vi "NI VeriStand - Create and Load Runtime Configuration File.vi"(6 "File Path":string, 7 "Version":string, 8 "Error in":errorcluster, 9 "Creator":string, 10 "Description":string, 11 "Name":string) -> (0 "Error out":errorcluster, 3 "Runtime Configuration Ref":refnum<k24>)   [LabVIEW 2026, in "NI_VS RuntimeConfigurationFile ScriptingAPI.lvlib"]
uses:
  NI_VS RuntimeConfigurationFile ScriptingAPI.lvlib
  NationalInstruments.VeriStand.SystemDefinitionAPI
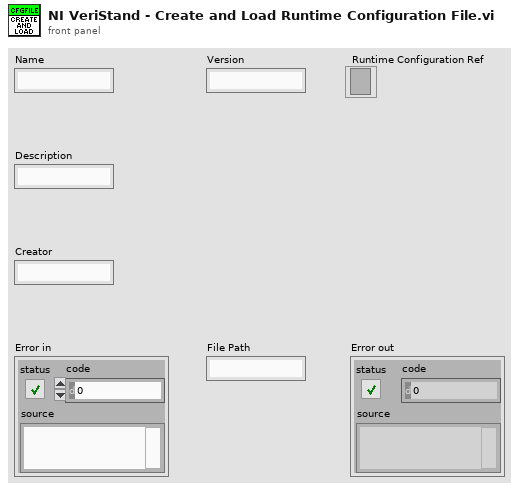
[diagram p1: front panel]
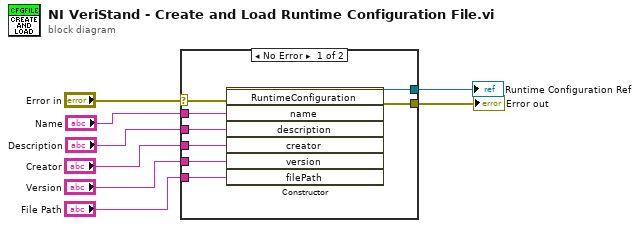
[diagram p0: block diagram]
diagram:
  n1 = case shown="No Error" "Error in" {
    selector: "Error in" -> [w16 w17]
    tunnel: "Name" -> [w14 _]
    tunnel: "Description" -> [w13 _]
    tunnel: "Creator" -> [w12 _]
    tunnel: "Version" -> [w11 _]
    tunnel: "File Path" -> [w10 _]
    tunnel: [w9 _] -> w1
    tunnel: [w15 w17] -> w8
    frame No Error {
      n2 = constructor class="RuntimeConfiguration"(error in=w16, "name"=w14, "description"=w13, "creator"=w12, "version"=w11, "filePath"=w10) -> (reference out=w9:refnum<k24>, error out=w15:errorcluster)  [unwired: 2 in, 6 out]
    }
    frame Error {
    }
  }
  "Runtime Configuration Ref" <- w1
  "Error out" <- w8
